vi "Recieve Message.vi"(8 "error in (no error)":errorcluster, 9 "Message":string, 10 "Sender":string, 11 "Message Reciever Interface in":refnum<class "Message Reciever Interface.lvclass">) -> (0 "error out":errorcluster, 3 "Message Reciever Interface out":refnum<class "Message Reciever Interface.lvclass">)   [LabVIEW 2020, in "Simple Chat.lvlib" / "Message Reciever Interface.lvclass"]
uses:
  Message Reciever Interface.lvclass
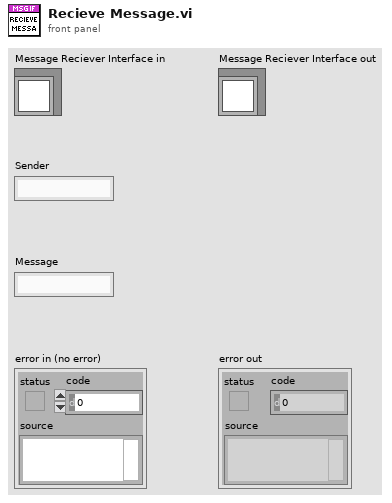
[diagram p1: front panel]
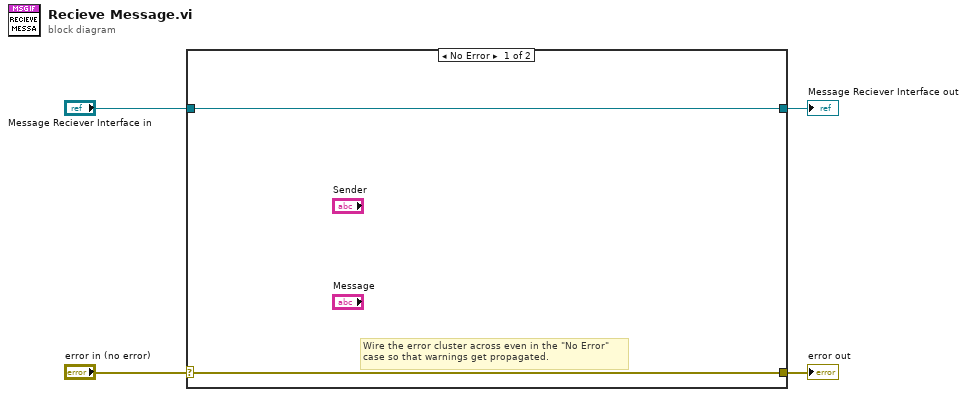
[diagram p0: block diagram]
diagram:
  n1 = case shown="No Error" "error in (no error)" {
    selector: "error in (no error)" -> [w5 w8]
    tunnel: [w5 w8] -> w3
    tunnel: [w6 w7] -> w1
    tunnel: "Message Reciever Interface in" -> [w6 w7]
    frame No Error {
      # "Wire the error cluster across even in the \"No Error\"\ncase so that warnings get propagated."
    }
    frame Error {
    }
  }
  "error out" <- w3
  "Message Reciever Interface out" <- w1
